vi "File explorer.vi"(0 "IP Address":string) -> ()   [LabVIEW 2017]
uses:
  <vilib>/FTP/ftp0.llb/FTP Session.ctl
  086dd945-d4c5-4c93-89ce-150d1d9cd8c6.vi
  <vilib>/Array/Sort 2D Array - Pop Stack.vi
  <vilib>/Array/Sort 2D Array - Push Stack.vi
  <vilib>/FTP/NI_FTP.lvlib
panel:
  out "Close":bool
  in  "Stop":bool
  in  "Directory Listing":i32(listbox)=-1
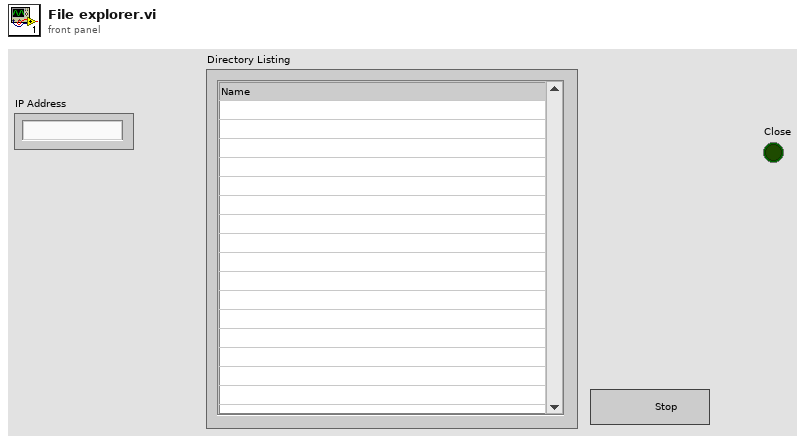
[diagram p1: front panel]
types:
  T1 = typedef "NI_FTP.lvlib/FTP Session.ctl" = refnum<k5>
  T2 = typedef "NI_FTP.lvlib/FTP File Info.ctl" = cluster{"type":enum16{"unknown", "file", "dir", "link"}, "permissions":string, "owner":string, "group":string, "size":i32, "date":string, "name":string, "link name":string}
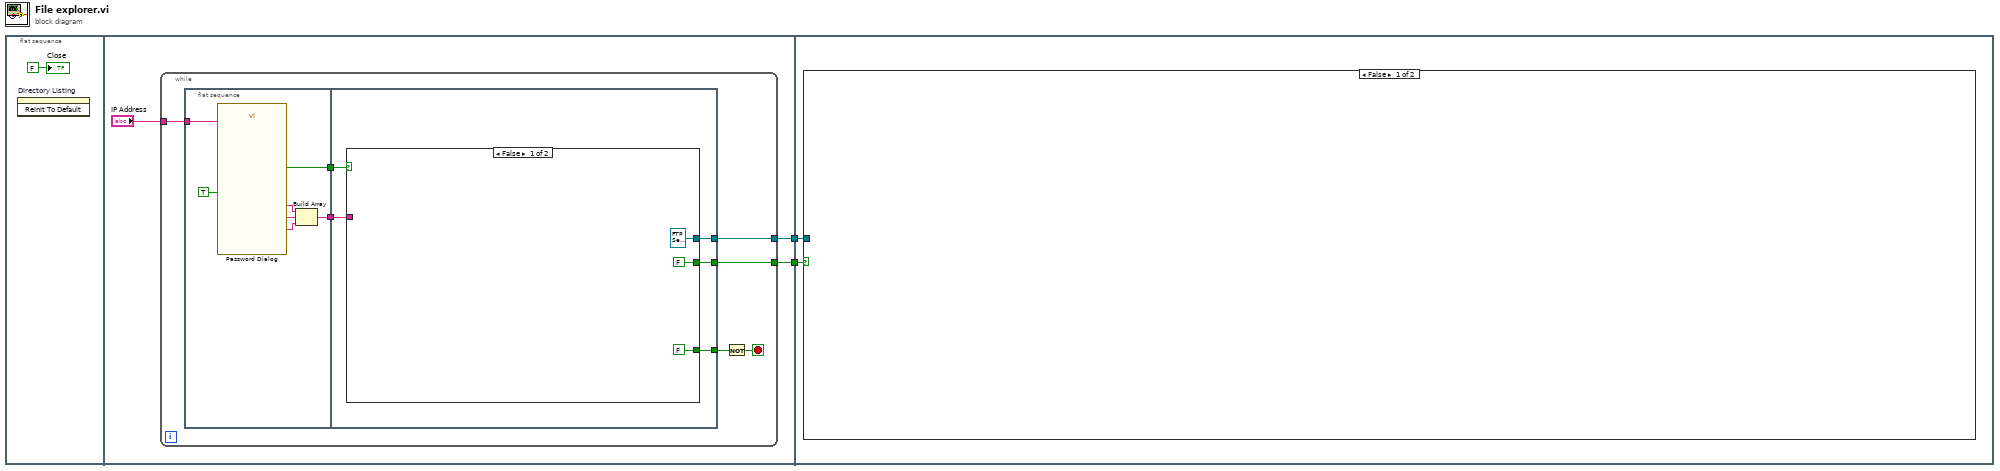
[diagram p0: block diagram]
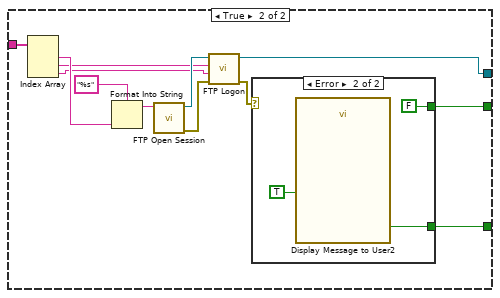
[diagram p2: hidden frame]
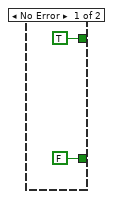
[diagram p3: hidden frame]
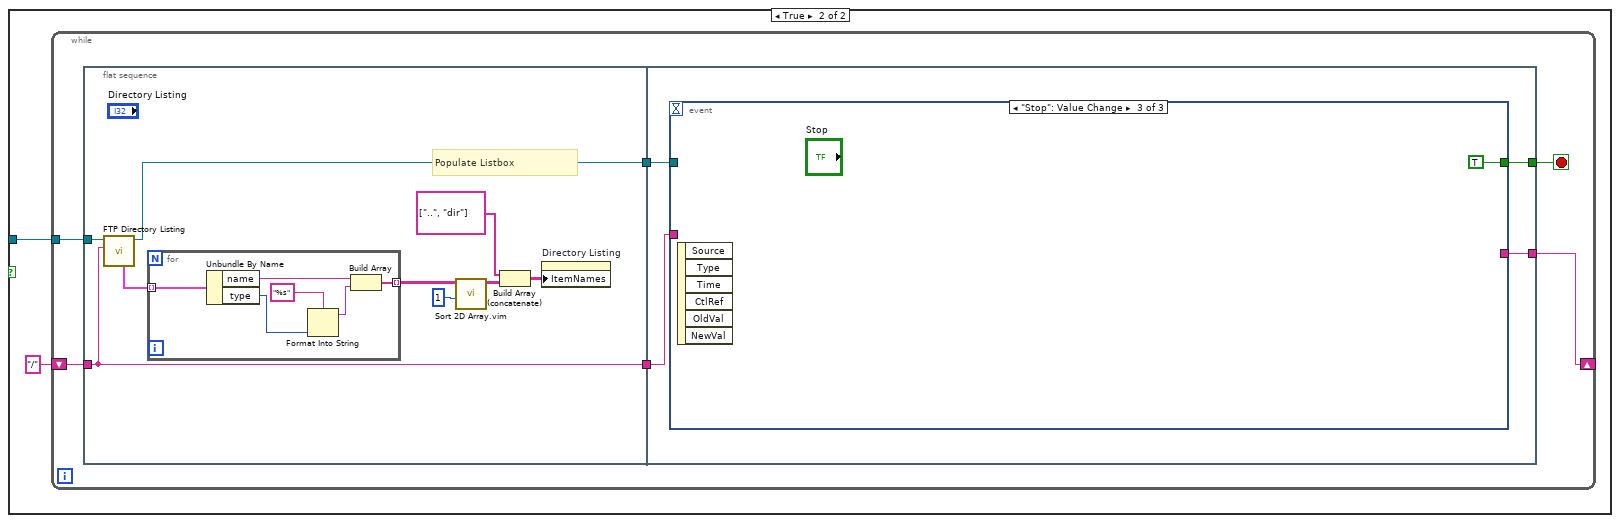
[diagram p4: hidden frame]
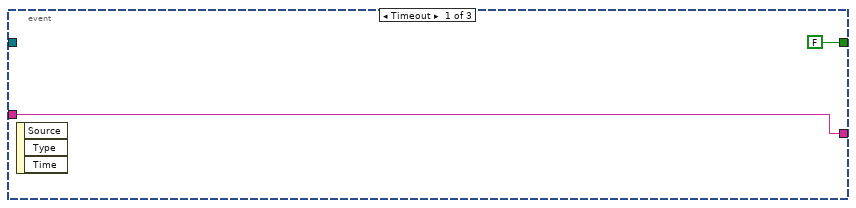
[diagram p5: hidden frame]
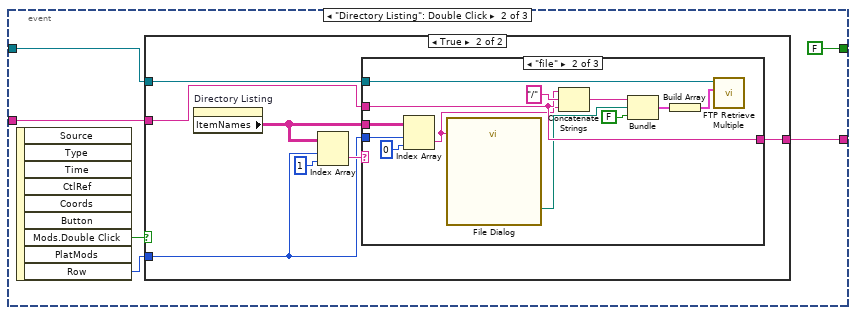
[diagram p6: hidden frame]
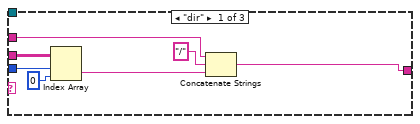
[diagram p8: hidden frame]
diagram:
  n1 = flat-sequence {
    tunnel: [w5] -> w2
    tunnel: [w4] -> w1
    tunnel: w2 -> [w47]
    tunnel: w1 -> [w46]
    frame #0 {
      n2 = invoke on="Directory Listing" class="MCListbox (strict)" method="Reinit To Default"() -> ()  [unwired: 3 in, 3 out]
      "Close" <- FALSE ("Close")
    }
    frame #1 {
      n3 = while {
        tunnel: "IP Address" -> [w12]
        tunnel: [w11] -> w5
        tunnel: [w7] -> w4
        stop <- w9 stop-if-true
        n4 = flat-sequence {
          tunnel: [w16] -> w13
          tunnel: w12 -> [w15]
          tunnel: [w14] -> w10
          tunnel: w13 -> [w25]
          tunnel: [w24] -> w8
          tunnel: [w23] -> w11
          tunnel: w10 -> [w22]
          tunnel: [w21] -> w7
          frame #0 {
            n5 = call "Password Dialog.vi"("Enable"=TRUE, "IP Placeholder"=w15) -> ("Password"=w17:string, "Username"=w18:string, "IP address"=w19:string, "OK"=w14:bool)  [unwired: 13 in, 1 out]
            n6 = Build Array(w19, w18, w17) -> (w16:string[])
          }
          frame #1 {
            n7 = case shown="False" w22 {
              tunnel: w25 -> [_ w40]
              tunnel: [FALSE ("Retry") w38] -> w24
              tunnel: [T1 refnum ("ftp session out") w30] -> w23
              tunnel: [FALSE ("Retry") w29] -> w21
              frame False {
              }
              frame True {
                n8 = Index Array(array=w40) -> (element #1=w39:string, element #2=w34:string, element #3=w33:string)  [unwired: 3 in]
                n9 = Format Into String(format string="%s", w39) -> (resulting string=w37:string)  [unwired: 2 in, 1 out]
                n10 = call <vilib>:"FTP Open Session.vi"("address"=w37) -> ("error out"=w35:errorcluster, "ftp session"=w36:T1)  [unwired: 7 in, 2 out]
                n11 = call <vilib>:"FTP Logon.vi"("error in (no error)"=w35, "password"=w33, "user"=w34, "ftp session"=w36) -> ("error out"=w31:errorcluster, "ftp session out"=w30:T1)  [unwired: 4 in, 2 out]
                n12 = case shown="Error" w31 {
                  tunnel: [FALSE ("Retry") w44] -> w38
                  tunnel: [TRUE FALSE] -> w29
                  frame No Error {
                  }
                  frame Error {
                    n13 = call "Display Message to User2"("Enable"=TRUE) -> ("Retry"=w44:bool)  [unwired: 9 in, 1 out]
                  }
                }
              }
            }
          }
        }
        n14 = Not(x=w8) -> (.not. x?=w9:bool)
      }
    }
    frame #2 {
      n15 = case shown="False" w46 {
        tunnel: w47 -> [_ w49]
        frame False {
        }
        frame True {
          n16 = while {
            tunnel: w49 -> [w55]
            shift-right: [w51] -> _
            shift-left: "/" -> [w54]
            stop <- w50 stop-if-true
            n17 = flat-sequence {
              tunnel: w55 -> [w64]
              tunnel: w54 -> [w56]
              tunnel: [w57] -> w53
              tunnel: [w56] -> w52
              tunnel: w53 -> [w74]
              tunnel: w52 -> [w73]
              tunnel: [w72] -> w51
              tunnel: [w71] -> w50
              frame #0 {
                # "Populate Listbox"
                n18 = call <vilib>:"FTP Directory Listing.vi"("directory path"=w56, "ftp session"=w64) -> ("ftp session out"=w57:T1, "dir list"=w63:T2[])  [unwired: 5 in, 3 out]
                n19 = for {
                  tunnel: w63 -> [w70] mode=indexing
                  tunnel: [w68] -> w60 mode=indexing
                  n20 = Unbundle By Name(w70) -> ("name"=w69:string, "type"=w67:enum16{"unknown", "file", "dir", "link"})
                  n21 = Format Into String(format string="%s", w67) -> (resulting string=w65:string)  [unwired: 2 in, 1 out]
                  n22 = Build Array(w69, w65) -> (w68:string[])
                }
                n23 = call "Sort 2D Array.vim"("index"=1, "2D array"=w60) -> ("sorted 2D array"=w59:string[][])  [unwired: 8 in, 1 out]
                n24 = Build Array (concatenate)(string[] ["..", "dir"], w59) -> (w62:string[][])
                n25 = property on="Directory Listing" class="MCListbox (strict)"("ItemNames"=w62) -> ()  [unwired: 2 in, 2 out]
              }
              frame #1 {
                n26 = event shown="[2] \"Stop\": Value Change" {
                  selector: _ -> [_ _ _]
                  dyn-events: _ -> [_ _ _]
                  timeout: _ -> [_ _ _]
                  tunnel: w73 -> [w76 w80 _]
                  tunnel: [w76 w79 _] -> w72
                  tunnel: w74 -> [_ w78 _]
                  tunnel: [FALSE FALSE TRUE] -> w71
                  event Timeout {
                    n27 = event-data() -> ()  [unwired: 1 in, 3 out]
                  }
                  event "Directory Listing": Double Click {
                    n28 = event-data() -> ("Mods.Double Click"=w82:bool, "Row"=w81:i32)  [unwired: 1 in, 7 out]
                    n29 = case shown="True" w82 {
                      tunnel: w80 -> [w83 w85]
                      tunnel: w81 -> [_ w86]
                      tunnel: [w83 w88] -> w79
                      tunnel: w78 -> [_ w84]
                      frame False {
                      }
                      frame True {
                        n30 = property on="Directory Listing" class="MCListbox (strict)"() -> ("ItemNames"=w87:string[][])  [unwired: 2 in, 2 out]
                        n31 = Index Array(array=w87, index (row)=w86, index (col)=1 ("disabled index (col)")) -> (element=w89:string)
                        n32 = case shown="\"file\"" w89 {
                          tunnel: [w96 w104 w110] -> w88
                          tunnel: w87 -> [w95 w107 _]
                          tunnel: w86 -> [w93 w108 _]
                          tunnel: w85 -> [w91 w104 w110]
                          tunnel: w84 -> [_ w106 _]
                          frame "dir" {
                            n33 = Index Array(array=w95, index (row)=w93, index (col)=0 ("disabled index (col)")) -> (element=w92:string)
                            n34 = Concatenate Strings(w91, "/" ("string"), w92) -> (w96:string)
                          }
                          frame "file" {
                            n35 = Index Array(array=w107, index (row)=w108, index (col)=0 ("disabled index (col)")) -> (element=w103:string)
                            n36 = call "File Dialog"("default name"=w103) -> ("selected path"=w101:path)  [unwired: 11 in, 3 out]
                            n37 = Concatenate Strings(w104, "/" ("string"), w103) -> (w102:string)
                            n38 = Bundle(w102, "selected path"=w101, FALSE) -> (w99:cluster{string, "selected path":path, bool})  [unwired: 1 in]
                            n39 = Build Array(w99) -> (w98:cluster{string, "selected path":path, bool}[])
                            n40 = call <vilib>:"FTP Retrieve Multiple.vi"("file specifications"=w98, "ftp session"=w106) -> ()  [unwired: 6 in, 4 out]
                          }
                          frame "link", "unknown", Default {
                          }
                        }
                      }
                    }
                  }
                  event "Stop": Value Change {
                    n41 = event-data() -> ()  [unwired: 1 in, 6 out]
                  }
                }
              }
            }
          }
        }
      }
    }
  }
